vi "Remove Create and Start Channels.vi"(8 "error in (no error)":errorcluster, 11 "Performanced XNET CAN Signal Logger in":refnum<class "Performanced XNET CAN Signal Logger.lvclass">) -> (0 "error out":errorcluster, 3 "Performanced XNET CAN Signal Logger out":refnum<class "Performanced XNET CAN Signal Logger.lvclass">)   [LabVIEW 2021, in "Performanced XNET CAN Signal Logger.lvlib" / "Performanced XNET CAN Signal Logger.lvclass"]
uses:
  Performanced XNET CAN Signal Logger.lvclass
  <vilib>/FlexLogger/SDK/PluginSDK.lvlibp/PEFClasses/SDK/Producer Channel/Producer Channel.lvclass
  C:/Program Files/National Instruments/LabVIEW 2021/vi.lib/FlexLogger/SDK/PluginSDK.lvlibp/PEFClasses/SDK/Channel/Channel.lvclass
  <vilib>/FlexLogger/SDK/PluginSDK.lvlibp/PEFClasses/SDK/Channel/Channel.lvclass
  Performanced XNET CAN Signal Logger.lvclass/Performanced XNET CAN Signal Logger.ctl
  XNET-CAN-Signal-Logger.lvlib
  <vilib>/FlexLogger/SDK/PluginSDK.lvlibp/PEFClasses/SDK/Plugin/Plugin.lvclass
  C:/Program Files/National Instruments/LabVIEW 2021/vi.lib/FlexLogger/SDK/PluginSDK.lvlibp/PEFClasses/SDK/Plugin/Plugin.lvclass
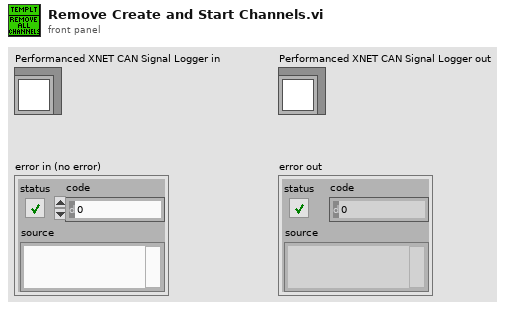
[diagram p1: front panel]
types:
  T1 = typedef "XNET-CAN-Signal-Logger.lvlib/Def-CAN Port Configuration.ctl" = cluster{"CAN Interface":refnum<k21>, "XNET Cluster":refnum<k21>, "#Signals":i32, "Sample Rate (Hz)":dbl}
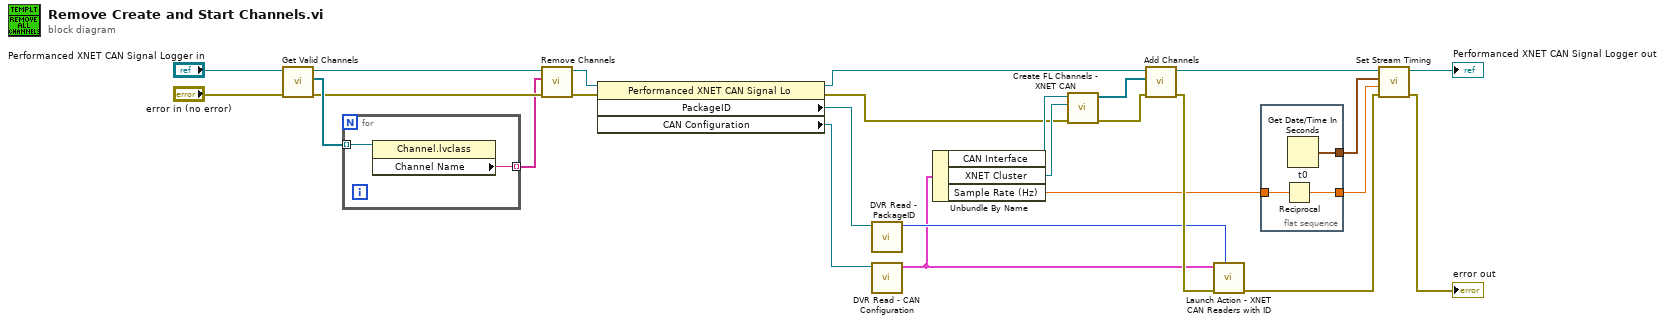
[diagram p0: block diagram]
diagram:
  n1 = call <vilib>:"Get Valid Channels.vi"("error in (no error)"="error in (no error)", "Plugin in"="Performanced XNET CAN Signal Logger in") -> ("error out"=w21:errorcluster, "Channels"=w23:refnum<class "Channel.lvclass">[], "Plugin out"=w22:refnum<class "Performanced XNET CAN Signal Logger.lvclass">)  [unwired: 7 in]
  n2 = for {
    tunnel: w23 -> [w28] mode=indexing
    tunnel: [w27] -> w20 mode=indexing
    n3 = property class="Channel.lvclass"(reference=w28) -> ("Channel Name"=w27:string)  [unwired: 1 in, 2 out]
  }
  n4 = call-dynamic "Remove Channels.vi"("error in (no error)"=w21, "Unique Channel Identifiers to Delete"=w20, "Plugin in"=w22) -> ("error out"=w16:errorcluster, "Plugin out"=w18:refnum<class "Performanced XNET CAN Signal Logger.lvclass">)  [unwired: 7 in]
  n5 = property class="Performanced XNET CAN Signal Lo"(reference=w18, error in=w16) -> (reference out=w25:refnum<class "Performanced XNET CAN Signal Logger.lvclass">, error out=w9:errorcluster, "PackageID"=w8:refnum<data-value>, "CAN Configuration"=w24:refnum<data-value>)
  n6 = call "DVR Read - PackageID.vi"("Data Value Reference in"=w8) -> ("PackageID"=w15:i32)  [unwired: 10 in]
  n7 = call "DVR Read - CAN Configuration.vi"("Data Value Reference in"=w24) -> ("CAN Port Configuration"=w11:T1)  [unwired: 10 in]
  n8 = Unbundle By Name(w11) -> ("CAN Interface"=w13:refnum<k21>, "XNET Cluster"=w14:refnum<k21>, "Sample Rate (Hz)"=w3:dbl)
  n9 = call "Create FL Channels - XNET CAN.vi"("error in (no error)"=w9, "XNET Cluster"=w14, "CAN Interface"=w13) -> ("error out"=w10:errorcluster, "Producer Channels"=w12:refnum<class "Producer Channel.lvclass">[])  [unwired: 6 in, 1 out]
  n10 = call <vilib>:"Add Channels.vi"("error in (no error)"=w10, "Channels"=w12, "Plugin in"=w25) -> ("error out"=w26:errorcluster, "Plugin out"=w5:refnum<class "Performanced XNET CAN Signal Logger.lvclass">)  [unwired: 7 in]
  n11 = call "Launch Action - XNET CAN Readers with ID.vi"("PackageID"=w15, "error in (no error)"=w26, "CAN Configuration"=w11) -> ("error out"=w2:errorcluster)  [unwired: 8 in]
  n12 = flat-sequence {
    tunnel: [w31] -> w6
    tunnel: [w30] -> w7
    tunnel: w3 -> [w29]
    frame #0 {
      n13 = Reciprocal(x=w29) -> (1/x=w30:dbl)
      n14 = Get Date/Time In Seconds "t0"() -> (seconds since 1Jan1904=w31:timestamp)
    }
  }
  n15 = call-dynamic "Set Stream Timing.vi"("error in (no error)"=w2, "dt(sec)"=w7, "Start Time"=w6, "Plugin in"=w5) -> ("error out"=→"error out":errorcluster, "Plugin out"=→"Performanced XNET CAN Signal Logger out":refnum<class "Performanced XNET CAN Signal Logger.lvclass">)  [unwired: 6 in]
